vi "Test Extended 64.vi"() -> ()   [LabVIEW 2019]
uses:
  <vilib>/addons/_JKI Toolkits/Caraya/classes/Assert/Assert Equal Value_Variant.vi
  <vilib>/addons/_JKI Toolkits/Caraya/classes/Assert/Assert Almost Equal_Float.vi
  <vilib>/addons/_JKI Toolkits/Caraya/classes/Assert/Assert.lvclass
  <vilib>/addons/_JKI Toolkits/Caraya/classes/Test/Test.lvclass
panel:
  out "error out":errorcluster
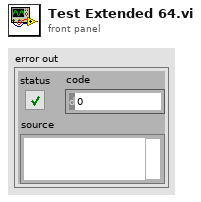
[diagram p1: front panel]
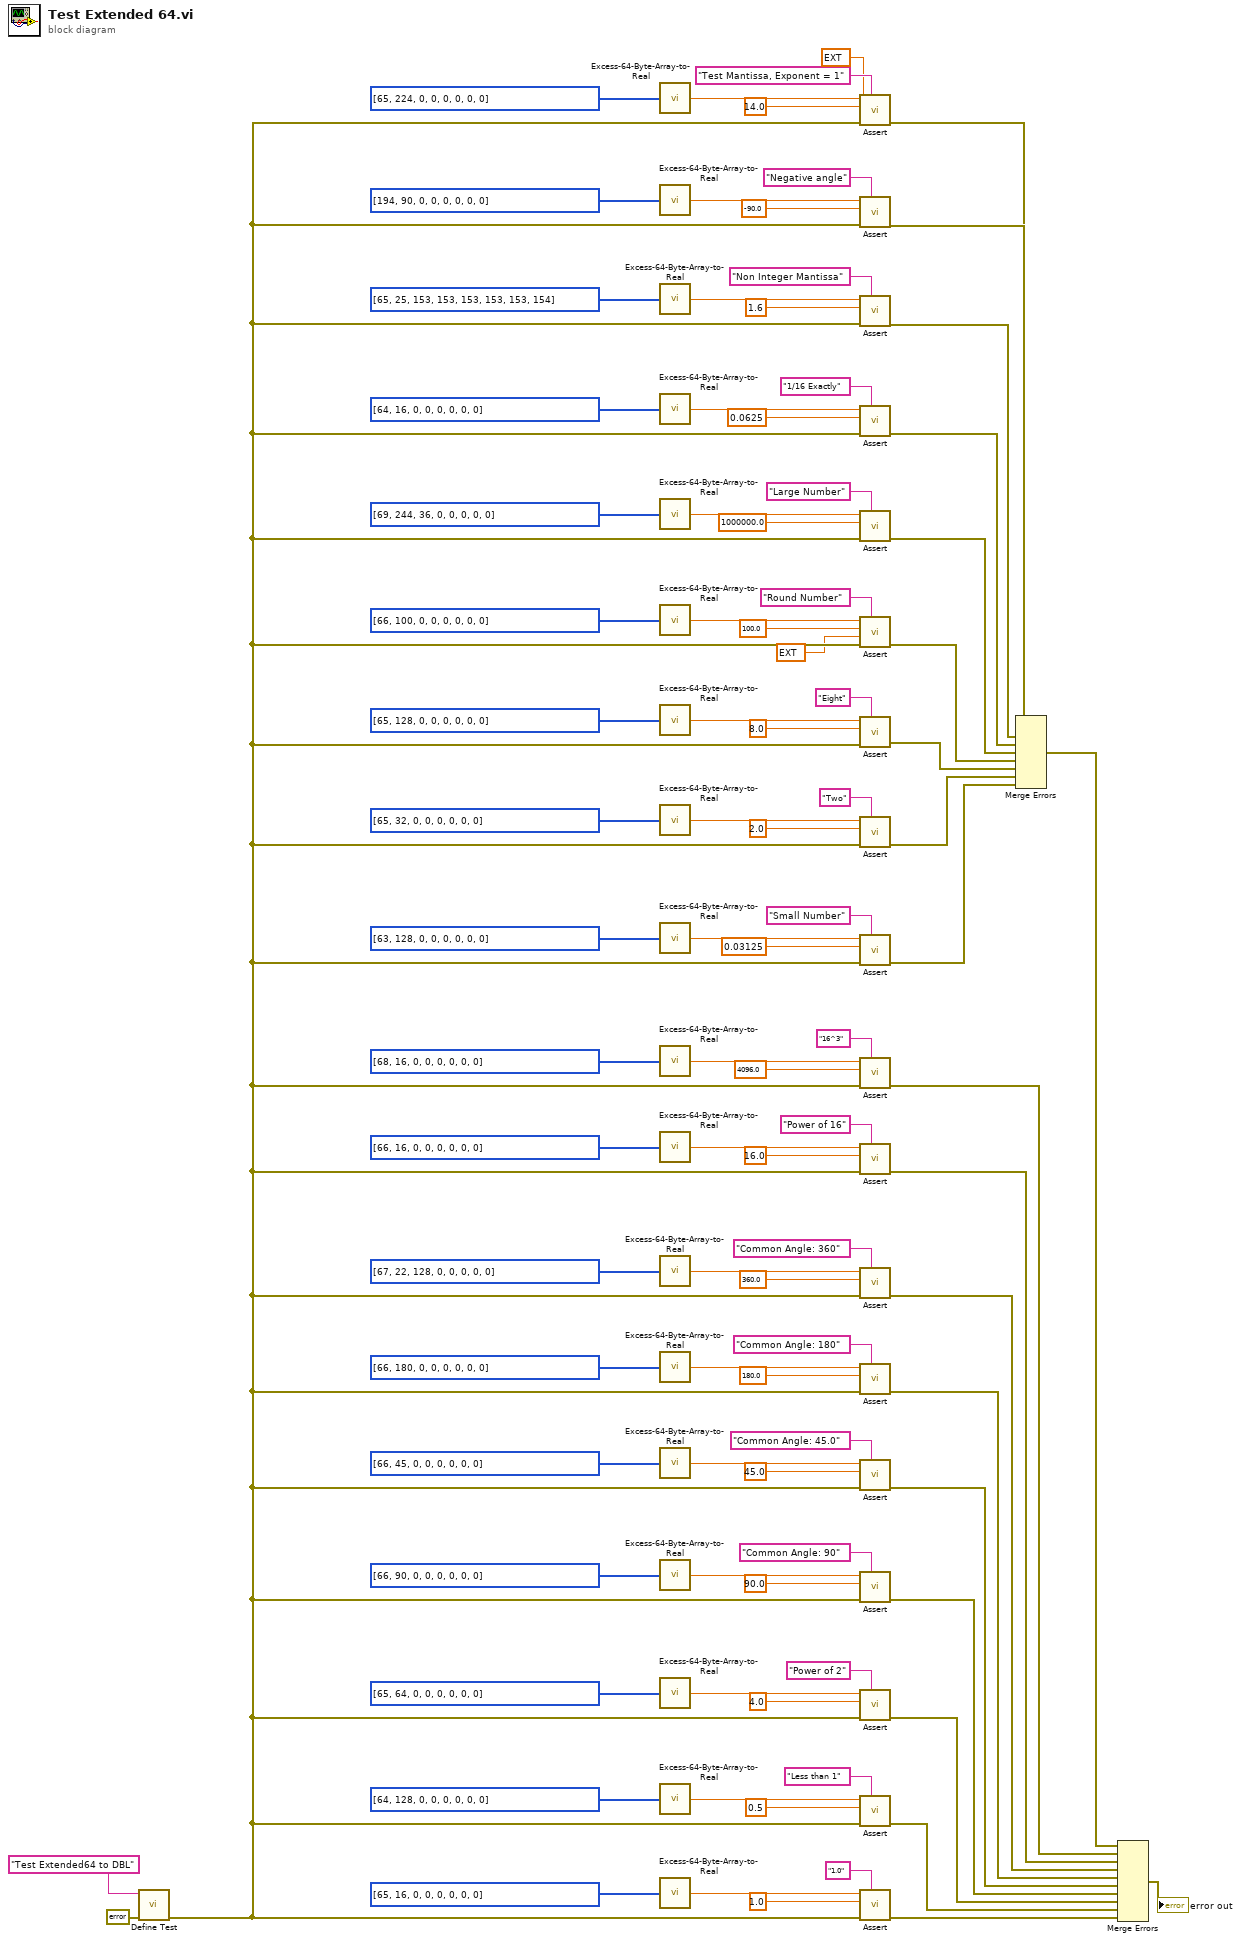
[diagram p0: block diagram]
diagram:
  n1 = call <vilib>:"Define Test.vi"("error in (no error)"=errorcluster {"status"=FALSE, "code"=0, "source"=""}, "Label (VI Title)"="Test Extended64 to DBL") -> ("error out"=w4:errorcluster)  [unwired: 8 in, 1 out]
  n2 = call "Excess-64-Byte-Array-to-Real.vi"("Byte array (4 or 8 bytes)"=u8[] [65, 224, 0, 0, 0, 0, 0, 0]) -> ("Real Number"=w6:dbl)  [unwired: 4 in]
  n3 = call "Excess-64-Byte-Array-to-Real.vi"("Byte array (4 or 8 bytes)"=u8[] [194, 90, 0, 0, 0, 0, 0, 0]) -> ("Real Number"=w12:dbl)  [unwired: 4 in]
  n4 = call "Excess-64-Byte-Array-to-Real.vi"("Byte array (4 or 8 bytes)"=u8[] [65, 25, 153, 153, 153, 153, 153, 154]) -> ("Real Number"=w16:dbl)  [unwired: 4 in]
  n5 = call "Excess-64-Byte-Array-to-Real.vi"("Byte array (4 or 8 bytes)"=u8[] [64, 16, 0, 0, 0, 0, 0, 0]) -> ("Real Number"=w22:dbl)  [unwired: 4 in]
  n6 = call "Excess-64-Byte-Array-to-Real.vi"("Byte array (4 or 8 bytes)"=u8[] [69, 244, 36, 0, 0, 0, 0, 0]) -> ("Real Number"=w31:dbl)  [unwired: 4 in]
  n7 = call "Excess-64-Byte-Array-to-Real.vi"("Byte array (4 or 8 bytes)"=u8[] [66, 100, 0, 0, 0, 0, 0, 0]) -> ("Real Number"=w36:dbl)  [unwired: 4 in]
  n8 = call "Excess-64-Byte-Array-to-Real.vi"("Byte array (4 or 8 bytes)"=u8[] [65, 128, 0, 0, 0, 0, 0, 0]) -> ("Real Number"=w39:dbl)  [unwired: 4 in]
  n9 = call "Excess-64-Byte-Array-to-Real.vi"("Byte array (4 or 8 bytes)"=u8[] [65, 32, 0, 0, 0, 0, 0, 0]) -> ("Real Number"=w44:dbl)  [unwired: 4 in]
  n10 = call "Excess-64-Byte-Array-to-Real.vi"("Byte array (4 or 8 bytes)"=u8[] [63, 128, 0, 0, 0, 0, 0, 0]) -> ("Real Number"=w47:dbl)  [unwired: 4 in]
  n11 = call "Excess-64-Byte-Array-to-Real.vi"("Byte array (4 or 8 bytes)"=u8[] [68, 16, 0, 0, 0, 0, 0, 0]) -> ("Real Number"=w53:dbl)  [unwired: 4 in]
  n12 = call "Excess-64-Byte-Array-to-Real.vi"("Byte array (4 or 8 bytes)"=u8[] [66, 16, 0, 0, 0, 0, 0, 0]) -> ("Real Number"=w57:dbl)  [unwired: 4 in]
  n13 = call "Excess-64-Byte-Array-to-Real.vi"("Byte array (4 or 8 bytes)"=u8[] [67, 22, 128, 0, 0, 0, 0, 0]) -> ("Real Number"=w63:dbl)  [unwired: 4 in]
  n14 = call "Excess-64-Byte-Array-to-Real.vi"("Byte array (4 or 8 bytes)"=u8[] [66, 180, 0, 0, 0, 0, 0, 0]) -> ("Real Number"=w67:dbl)  [unwired: 4 in]
  n15 = call "Excess-64-Byte-Array-to-Real.vi"("Byte array (4 or 8 bytes)"=u8[] [66, 45, 0, 0, 0, 0, 0, 0]) -> ("Real Number"=w73:dbl)  [unwired: 4 in]
  n16 = call "Excess-64-Byte-Array-to-Real.vi"("Byte array (4 or 8 bytes)"=u8[] [66, 90, 0, 0, 0, 0, 0, 0]) -> ("Real Number"=w78:dbl)  [unwired: 4 in]
  n17 = call "Excess-64-Byte-Array-to-Real.vi"("Byte array (4 or 8 bytes)"=u8[] [65, 64, 0, 0, 0, 0, 0, 0]) -> ("Real Number"=w84:dbl)  [unwired: 4 in]
  n18 = call "Excess-64-Byte-Array-to-Real.vi"("Byte array (4 or 8 bytes)"=u8[] [64, 128, 0, 0, 0, 0, 0, 0]) -> ("Real Number"=w89:dbl)  [unwired: 4 in]
  n19 = call "Excess-64-Byte-Array-to-Real.vi"("Byte array (4 or 8 bytes)"=u8[] [65, 16, 0, 0, 0, 0, 0, 0]) -> ("Real Number"=w91:dbl)  [unwired: 4 in]
  n20 = call-poly <vilib>:"Assert.vi"("Label"="Test Mantissa, Exponent = 1" ("Label (VI Title)"), "error in (no error)"=w4, "Tolerance"=ext 0.00000100000000000000000004, "Actual"=14.0 ("Real Number"), "Expected"=w6) -> ("error out"=w3:errorcluster)  [unwired: 5 in, 1 out]
  n21 = call-poly <vilib>:"Assert.vi"("Label"="Negative angle" ("Label (VI Title)"), "error in (no error)"=w4, "Actual"=-90.0 ("Real Number"), "Expected"=w12) -> ("error out"=w9:errorcluster)  [unwired: 6 in, 1 out]
  n22 = call-poly <vilib>:"Assert.vi"("Label"="Non Integer Mantissa" ("Label (VI Title)"), "error in (no error)"=w4, "Actual"=1.6 ("Real Number"), "Expected"=w16) -> ("error out"=w14:errorcluster)  [unwired: 6 in, 1 out]
  n23 = call-poly <vilib>:"Assert.vi"("Label"="1/16 Exactly" ("Label (VI Title)"), "error in (no error)"=w4, "Actual"=0.0625 ("Real Number"), "Expected"=w22) -> ("error out"=w19:errorcluster)  [unwired: 6 in, 1 out]
  n24 = call-poly <vilib>:"Assert.vi"("Label"="Large Number" ("Label (VI Title)"), "error in (no error)"=w4, "Actual"=1000000.0 ("Real Number"), "Expected"=w31) -> ("error out"=w29:errorcluster)  [unwired: 6 in, 1 out]
  n25 = call-poly <vilib>:"Assert.vi"("Label"="Round Number" ("Label (VI Title)"), "error in (no error)"=w4, "Tolerance"=ext 0.00000100000000000000000004, "Actual"=100.0 ("Real Number"), "Expected"=w36) -> ("error out"=w28:errorcluster)  [unwired: 5 in, 1 out]
  n26 = call-poly <vilib>:"Assert.vi"("Label"="Eight" ("Label (VI Title)"), "error in (no error)"=w4, "Actual"=8.0 ("Real Number"), "Expected"=w39) -> ("error out"=w24:errorcluster)  [unwired: 6 in, 1 out]
  n27 = call-poly <vilib>:"Assert.vi"("Label"="Two" ("Label (VI Title)"), "error in (no error)"=w4, "Actual"=2.0 ("Real Number"), "Expected"=w44) -> ("error out"=w27:errorcluster)  [unwired: 6 in, 1 out]
  n28 = call-poly <vilib>:"Assert.vi"("Label"="Small Number" ("Label (VI Title)"), "error in (no error)"=w4, "Actual"=0.03125 ("Real Number"), "Expected"=w47) -> ("error out"=w26:errorcluster)  [unwired: 6 in, 1 out]
  n29 = call-poly <vilib>:"Assert.vi"("Label"="16^3" ("Label (VI Title)"), "error in (no error)"=w4, "Actual"=4096.0 ("Real Number"), "Expected"=w53) -> ("error out"=w50:errorcluster)  [unwired: 6 in, 1 out]
  n30 = call-poly <vilib>:"Assert.vi"("Label"="Power of 16" ("Label (VI Title)"), "error in (no error)"=w4, "Actual"=16.0 ("Real Number"), "Expected"=w57) -> ("error out"=w55:errorcluster)  [unwired: 6 in, 1 out]
  n31 = call-poly <vilib>:"Assert.vi"("Label"="Common Angle: 360" ("Label (VI Title)"), "error in (no error)"=w4, "Actual"=360.0 ("Real Number"), "Expected"=w63) -> ("error out"=w60:errorcluster)  [unwired: 6 in, 1 out]
  n32 = call-poly <vilib>:"Assert.vi"("Label"="Common Angle: 180" ("Label (VI Title)"), "error in (no error)"=w4, "Actual"=180.0 ("Real Number"), "Expected"=w67) -> ("error out"=w65:errorcluster)  [unwired: 6 in, 1 out]
  n33 = call-poly <vilib>:"Assert.vi"("Label"="Common Angle: 45.0" ("Label (VI Title)"), "error in (no error)"=w4, "Actual"=45.0 ("Real Number"), "Expected"=w73) -> ("error out"=w70:errorcluster)  [unwired: 6 in, 1 out]
  n34 = call-poly <vilib>:"Assert.vi"("Label"="Common Angle: 90" ("Label (VI Title)"), "error in (no error)"=w4, "Actual"=90.0 ("Real Number"), "Expected"=w78) -> ("error out"=w76:errorcluster)  [unwired: 6 in, 1 out]
  n35 = call-poly <vilib>:"Assert.vi"("Label"="Power of 2" ("Label (VI Title)"), "error in (no error)"=w4, "Actual"=4.0 ("Real Number"), "Expected"=w84) -> ("error out"=w81:errorcluster)  [unwired: 6 in, 1 out]
  n36 = call-poly <vilib>:"Assert.vi"("Label"="Less than 1" ("Label (VI Title)"), "error in (no error)"=w4, "Actual"=0.5 ("Real Number"), "Expected"=w89) -> ("error out"=w87:errorcluster)  [unwired: 6 in, 1 out]
  n37 = call-poly <vilib>:"Assert.vi"("Label"="1.0" ("Label (VI Title)"), "error in (no error)"=w4, "Actual"=1.0 ("Real Number"), "Expected"=w91) -> ("error out"=w96:errorcluster)  [unwired: 6 in, 1 out]
  n38 = Merge Errors(w3, w9, w14, w19, w29, w28, w24, w27, w26) -> (w25:errorcluster)
  n39 = Merge Errors(w25, w50, w55, w60, w65, w70, w76, w81, w87, w96) -> (→"error out":errorcluster)
